vi "Routines.Compile.vi"(8 "error in (no error)":errorcluster, 11 "Section Ref in":T4 format="%.0x") -> (0 "error out":errorcluster, 2 "Settings":T1 {"Signal.Cmd.Refs"."Signal Refs" format="%.0x"; "Signal.Cmd.Info"."Signals"."Byte Order" items=["Little Endian", "Big Endian"]; "Signal.Cmd.Info"."Signals"."Data Type" items=["Signed", "Unsigned", "IEEE Float"]; "Settings.Refs"."Signal Refs" format="%.0x"; "Signal.Resp.Refs"."Signal Refs" format="%.0x"; "Signal.Resp.Info"."Signals"."Byte Order" items=["Little Endian", "Big Endian"]; "Signal.Resp.Info"."Signals"."Data Type" items=["Signed", "Unsigned", "IEEE Float"]; "Trigger.Refs"."Signal Refs" format="%.0x"; "Status.Refs"."Signal Refs" format="%.0x"}, 3 "Section Ref out":T4 format="%.0x")   [LabVIEW 2019, in "Diagnostics Addon System Explorer.lvlib"]
uses:
  Diagnostics Addon System Explorer.lvlib
  <vilib>/NI VeriStand/Custom Device API/Custom Device Item Ref.ctl
  Types/Service.Export.ctl
  Types/Frame.Ref.ctl
  Addon Shared/Types/Type.ctl
  Addon Shared/Types/Frame.Compile.ctl
  Addon Shared/Types/Signal.ctl
  Types/FG.Action.ctl
  Signal.FG.vi
  Frame.GetSignalRefs.vi
  Addon Shared/SubVIs/Constants.vi
  <vilib>/NI VeriStand/Custom Device Tools/Custom Device Utility Library/NI VeriStand - Search for Item by GUID.vi
  <vilib>/NI/NI VeriStand Advanced SysDef API/SysDef API/SysDef.Property.Set.vi
  <vilib>/NI/NI VeriStand Advanced SysDef API/_SubVIs/SysDef.Property.Set.U32.vi
  <vilib>/NI VeriStand/Custom Device API/NI VeriStand - Get Item Property.vi
  <vilib>/NI VeriStand/Custom Device API/Get Item Property (U32).vi
  <vilib>/NI VeriStand/Custom Device Tools/Custom Device Utility Library/NI VeriStand - Search for Item by Name.vi
  <vilib>/NI VeriStand/Custom Device API/NI VeriStand - Get Item Data.vi
  <vilib>/NI/NI VeriStand Advanced SysDef API/_SubVIs/SysDef.Property.Set.DBL.vi
  <vilib>/NI/NI VeriStand Advanced SysDef API/_SubVIs/SysDef.Property.Set.String.vi
  <vilib>/NI VeriStand/Custom Device API/Get Item Property (Double).vi
  <vilib>/NI VeriStand/Custom Device API/Get Item Property (String).vi
  <vilib>/NI VeriStand/Custom Device API/NI VeriStand - Get Custom Device Channel Data.vi
  <vilib>/NI VeriStand/Custom Device Tools/Custom Device Utility Library/Custom Device Utility Library.lvlib
  <vilib>/NI VeriStand/Custom Device API/Custom Device API.lvlib
  Addon Shared/Diagnostics Addon Shared.lvlib
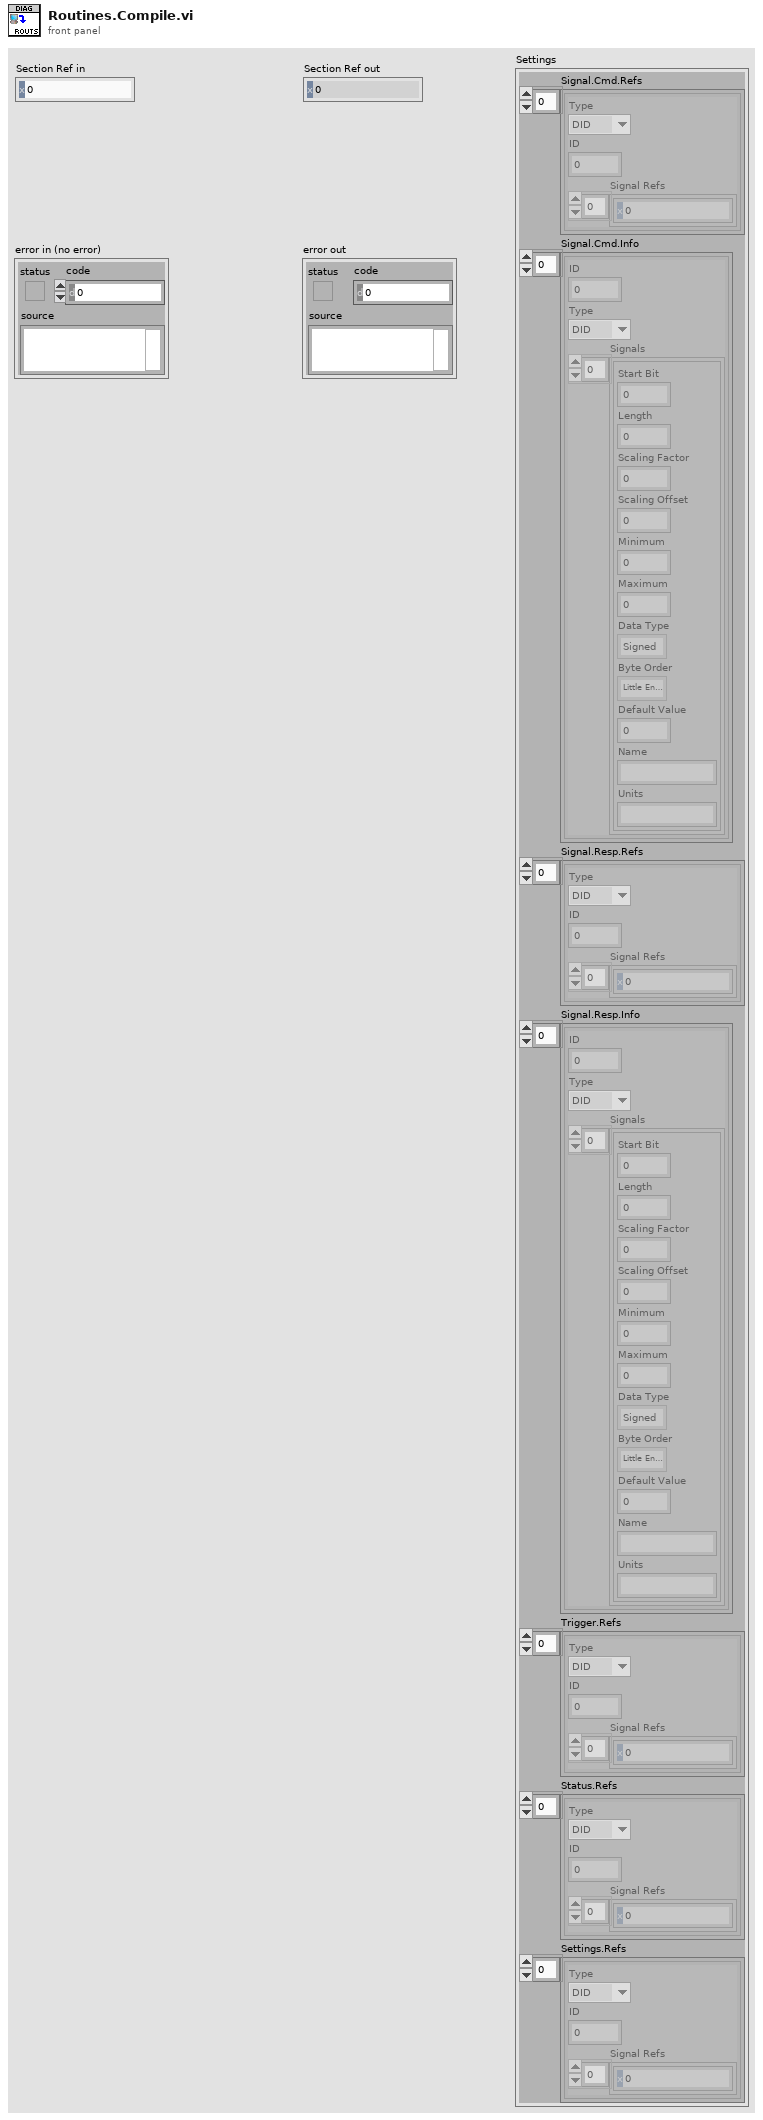
[diagram p1: front panel]
types:
  T1 = typedef "Diagnostics Addon System Explorer.lvlib/Service.Export.ctl" = cluster{"Signal.Cmd.Refs":T2[], "Signal.Cmd.Info":T5[], "Signal.Resp.Refs":T2[], "Signal.Resp.Info":T5[], "Trigger.Refs":T2[], "Status.Refs":T2[], "Settings.Refs":T2[]}
  T2 = typedef "Diagnostics Addon System Explorer.lvlib/Frame.Ref.ctl" = cluster{"Type":T3, "ID":u32, "Signal Refs":T4[]}
  T3 = typedef "Diagnostics Addon Shared.lvlib/Type.ctl" = enum16{"DID", "CDID", "PID", "CPID", "Read Memory", "Write Memory", "IO Control", "Routine Start", "Routine Request", "Routine Stop", "User Defined", "DTC Control", "Clear DTCs", "Read DTCs", "Start DTCs", "DTC Change Count", "Tester Present", "Unlock ECU", "Reset ECU", "Diag Session Control", "Communication Control", "DPID Control", "Poll Control", "Diag CAN Control"}
  T4 = typedef "Custom Device API.lvlib/Custom Device Item Ref.ctl" = u64
  T5 = typedef "Diagnostics Addon Shared.lvlib/Frame.Compile.ctl" = cluster{"ID":u32, "Type":T3, "Signals":T6[]}
  T6 = typedef "Diagnostics Addon Shared.lvlib/Signal.ctl" = cluster{"Start Bit":u32, "Length":u32, "Scaling Factor":dbl, "Scaling Offset":dbl, "Minimum":dbl, "Maximum":dbl, "Data Type":u32, "Byte Order":u32, "Default Value":dbl, "Name":string, "Units":string}
  T7 = typedef "Diagnostics Addon System Explorer.lvlib/FG.Action.ctl" = enum16{"Get", "Set"}
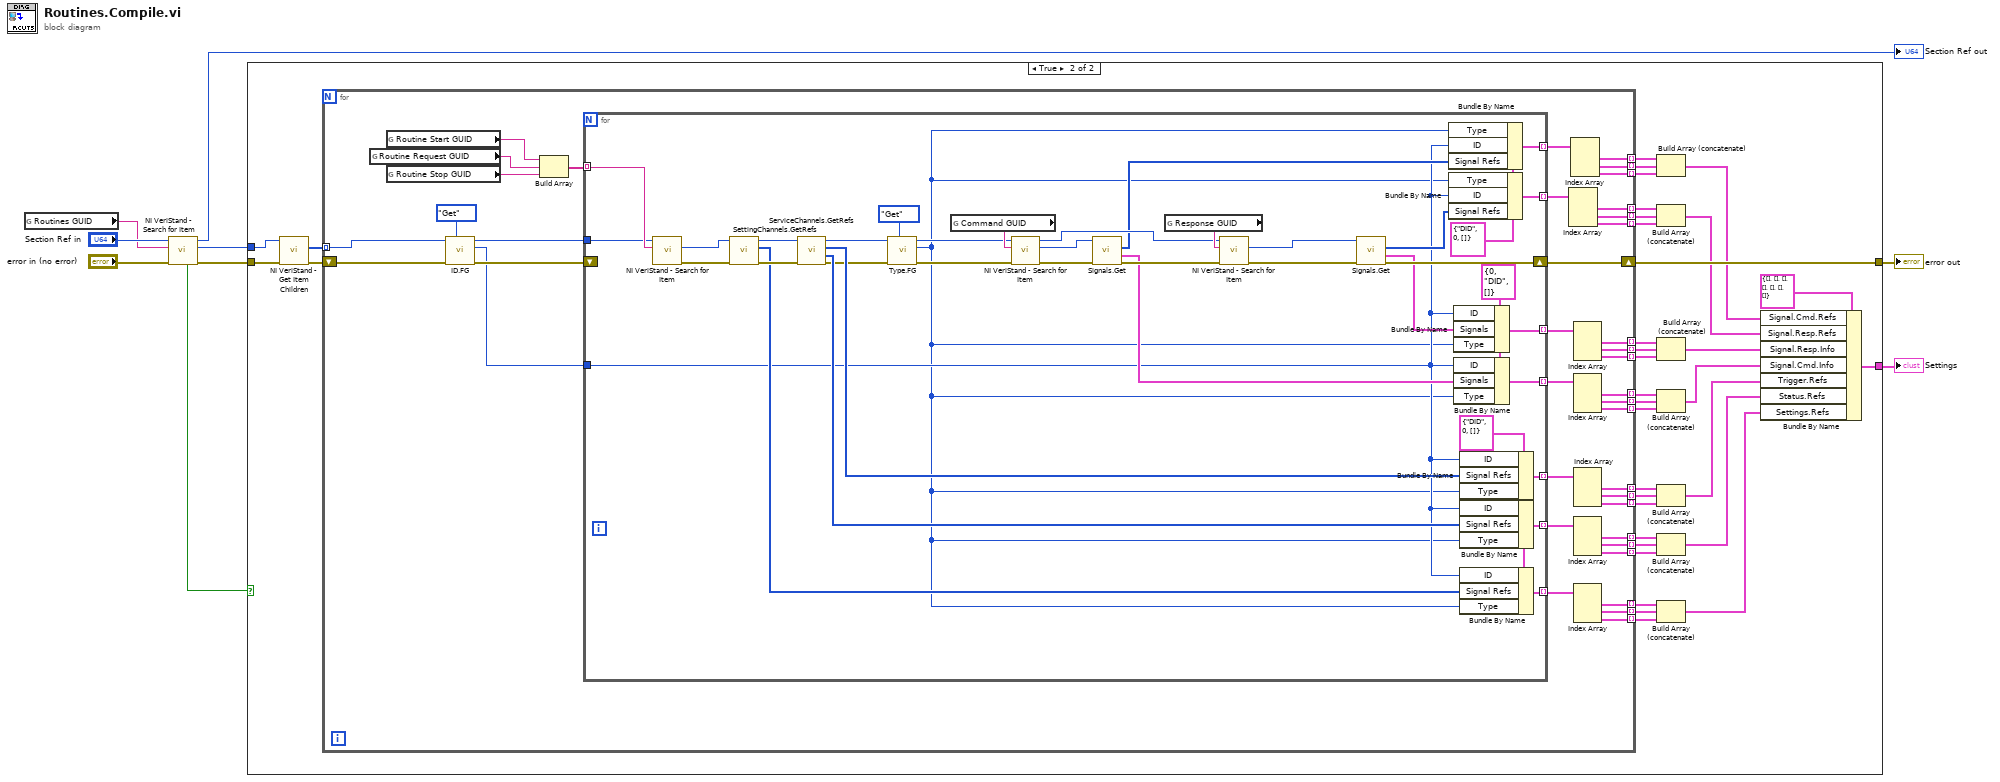
[diagram p0: block diagram]
diagram:
  n1 = global read "Constants.vi" "Routines GUID"() -> (w2:string)
  n2 = call-poly <vilib>:"NI VeriStand - Search for Item.vi"("error in"="error in (no error)", "Item GUID"=w2, "Section Ref in"="Section Ref in") -> ("error out"=w4:errorcluster, "Item Ref"=w5:T4, "Section Ref out"=→"Section Ref out":T4, "Found"=w3:bool)  [unwired: 5 in]
  n3 = case shown="True" w3 {
    tunnel: [w10 w45] -> w8
    tunnel: w5 -> [_ w42]
    tunnel: w4 -> [w10 w41]
    tunnel: [_ w23] -> w1
    frame False {
    }
    frame True {
      n4 = call <vilib>:"NI VeriStand - Get Item Children.vi"("error in (no error)"=w41, "Item Ref in"=w42) -> ("error out"=w43:errorcluster, "Child Refs"=w44:T4[])  [unwired: 6 in, 2 out]
      n5 = for {
        shift-right: [w76] -> w45
        shift-left: w43 -> [w59]
        tunnel: w44 -> [w58] mode=indexing
        tunnel: [w74] -> w31 mode=indexing
        tunnel: [w73] -> w29 mode=indexing
        tunnel: [w72] -> w28 mode=indexing
        tunnel: [w70] -> w30 mode=indexing
        tunnel: [w69] -> w26 mode=indexing
        tunnel: [w68] -> w25 mode=indexing
        tunnel: [w66] -> w40 mode=indexing
        tunnel: [w65] -> w39 mode=indexing
        tunnel: [w64] -> w38 mode=indexing
        tunnel: [w63] -> w35 mode=indexing
        tunnel: [w62] -> w34 mode=indexing
        tunnel: [w61] -> w33 mode=indexing
        tunnel: [w52] -> w17 mode=indexing
        tunnel: [w53] -> w19 mode=indexing
        tunnel: [w54] -> w20 mode=indexing
        tunnel: [w55] -> w18 mode=indexing
        tunnel: [w56] -> w21 mode=indexing
        tunnel: [w57] -> w22 mode=indexing
        tunnel: [w48] -> w14 mode=indexing
        tunnel: [w47] -> w13 mode=indexing
        tunnel: [w46] -> w12 mode=indexing
        n6 = global read "Constants.vi" "Routine Request GUID"() -> (w81:string)
        n7 = global read "Constants.vi" "Routine Start GUID"() -> (w83:string)
        n8 = global read "Constants.vi" "Routine Stop GUID"() -> (w80:string)
        n9 = call "ID.FG.vi"("Action"=FG.Action."Get", "error in (no error)"=w59, "Device Item Ref in"=w58) -> ("error out"=w78:errorcluster, "ID"=w60:u32, "Device Item Ref out"=w79:T4)  [unwired: 6 in]
        n10 = Build Array(w83, w81, w80) -> (w82:string[])
        n11 = for {
          tunnel: w82 -> [w123] mode=indexing
          tunnel: w79 -> [w104]
          shift-right: [w118] -> w76
          shift-left: w78 -> [_]
          tunnel: w60 -> [w95]
          tunnel: [w114] -> w75 mode=indexing
          tunnel: [w113] -> w71 mode=indexing
          tunnel: [w111] -> w77 mode=indexing
          tunnel: [w108] -> w67 mode=indexing
          tunnel: [w105] -> w51 mode=indexing
          tunnel: [w98] -> w50 mode=indexing
          tunnel: [w99] -> w49 mode=indexing
          w97 = T2 {"Type"=enum."DID", "ID"=0, "Signal Refs"=[]} ("cluster")
          w109 = T2 {"Type"=enum."DID", "ID"=0, "Signal Refs"=[]} ("Status.Cmd")
          w117 = T5 {"ID"=0, "Type"=enum."DID", "Signals"=[]} ("PID In")
          n12 = call-poly <vilib>:"NI VeriStand - Search for Item.vi"("Item GUID"=w123, "Section Ref in"=w104) -> ("error out"=w101:errorcluster, "Item Ref"=w103:T4)  [unwired: 6 in, 2 out]
          n13 = call "SettingChannels.GetRefs.vi"("error in (no error)"=w101, "Item Ref in"=w103) -> ("error out"=w100:errorcluster, "Settings"=w96:T4[], "Section Ref out"=w102:T4)  [unwired: 7 in]
          n14 = call "ServiceChannels.GetRefs.vi"("error in (no error)"=w100, "Item Ref in"=w102) -> ("error out"=w91:errorcluster, "Status"=w106:T4[], "Trigger"=w107:T4[], "Section Ref out"=w89:T4)  [unwired: 6 in]
          n15 = call "Type.FG.vi"("Action"=FG.Action."Get", "error in (no error)"=w91, "Device Item Ref in"=w89) -> ("error out"=w90:errorcluster, "Type"=w85:T3, "Device Item Ref out"=w88:T4)  [unwired: 6 in]
          n16 = global read "Constants.vi" "Command GUID"() -> (w122:string)
          n17 = call-poly <vilib>:"NI VeriStand - Search for Item.vi"("error in"=w90, "Item GUID"=w122, "Section Ref in"=w88) -> ("error out"=w94:errorcluster, "Item Ref"=w93:T4, "Section Ref out"=w120:T4)  [unwired: 5 in, 1 out]
          n18 = call "Signals.Get.vi"("error in (no error)"=w94, "Device Item Ref out"=w93) -> ("error out"=w119:errorcluster, "Parameters"=w116:T6[], "Child Refs"=w110:T4[])  [unwired: 6 in, 1 out]
          n19 = global read "Constants.vi" "Response GUID"() -> (w121:string)
          n20 = call-poly <vilib>:"NI VeriStand - Search for Item.vi"("error in"=w119, "Item GUID"=w121, "Section Ref in"=w120) -> ("error out"=w86:errorcluster, "Item Ref"=w87:T4)  [unwired: 5 in, 2 out]
          n21 = call "Signals.Get.vi"("error in (no error)"=w86, "Device Item Ref out"=w87) -> ("error out"=w118:errorcluster, "Parameters"=w115:T6[], "Child Refs"=w112:T4[])  [unwired: 6 in, 1 out]
          n22 = Bundle By Name(cluster=w109, "Type"=w85, "ID"=w95, "Signal Refs"=w110) -> (w108:T2)
          n23 = Bundle By Name(cluster=w109, "Type"=w85, "ID"=w95, "Signal Refs"=w112) -> (w111:T2)
          n24 = Bundle By Name(cluster=w117, "ID"=w95, "Signals"=w115, "Type"=w85) -> (w114:T5)
          n25 = Bundle By Name(cluster=w117, "ID"=w95, "Signals"=w116, "Type"=w85) -> (w113:T5)
          n26 = Bundle By Name(cluster=w97, "ID"=w95, "Signal Refs"=w107, "Type"=w85) -> (w105:T2)
          n27 = Bundle By Name(cluster=w97, "ID"=w95, "Signal Refs"=w106, "Type"=w85) -> (w98:T2)
          n28 = Bundle By Name(cluster=w97, "ID"=w95, "Signal Refs"=w96, "Type"=w85) -> (w99:T2)
        }
        n29 = Index Array(array=w77) -> (element #1=w63:T2, element #2=w62:T2, element #3=w61:T2)  [unwired: 3 in]
        n30 = Index Array(array=w67) -> (element #1=w66:T2, element #2=w65:T2, element #3=w64:T2)  [unwired: 3 in]
        n31 = Index Array(array=w75) -> (element #1=w74:T5, element #2=w73:T5, element #3=w72:T5)  [unwired: 3 in]
        n32 = Index Array(array=w71) -> (element #1=w70:T5, element #2=w69:T5, element #3=w68:T5)  [unwired: 3 in]
        n33 = Index Array(array=w51) -> (element #1=w52:T2, element #2=w53:T2, element #3=w54:T2)  [unwired: 3 in]
        n34 = Index Array(array=w50) -> (element #1=w55:T2, element #2=w56:T2, element #3=w57:T2)  [unwired: 3 in]
        n35 = Index Array(array=w49) -> (element #1=w48:T2, element #2=w47:T2, element #3=w46:T2)  [unwired: 3 in]
      }
      n36 = Build Array (concatenate)(w40, w39, w38) -> (w36:T2[])
      n37 = Build Array (concatenate)(w35, w34, w33) -> (w32:T2[])
      n38 = Build Array (concatenate)(w31, w29, w28) -> (w27:T5[])
      n39 = Build Array (concatenate)(w30, w26, w25) -> (w24:T5[])
      n40 = Build Array (concatenate)(w17, w19, w20) -> (w16:T2[])
      n41 = Build Array (concatenate)(w18, w21, w22) -> (w15:T2[])
      n42 = Build Array (concatenate)(w14, w13, w12) -> (w11:T2[])
      n43 = Bundle By Name(cluster=T1 {"Signal.Cmd.Refs"=[], "Signal.Cmd.Info"=[], "Signal.Resp.Refs"=[], "Signal.Resp.Info"=[], "Trigger.Refs"=[], "Status.Refs"=[], "Settings.Refs"=[]} ("Settings"), "Signal.Cmd.Refs"=w36, "Signal.Resp.Refs"=w32, "Signal.Resp.Info"=w27, "Signal.Cmd.Info"=w24, "Trigger.Refs"=w16, "Status.Refs"=w15, "Settings.Refs"=w11) -> (w23:T1)
    }
  }
  "error out" <- w8
  "Settings" <- w1
